vi "MENU8.vi"   [LabVIEW 2010, in "Lazyboots Menu Tool Launch.lvlib"]
uses:
  _Library/Lazyboots Menu Tool Launch.lvlib
  <vilib>/Utility/config.llb/Read Key (String).vi
  <vilib>/Utility/config.llb/NI_LVConfig.lvlib
panel:
  # "Launching..."
types:
  T1 = enum32{"Invalid", "Standard", "Closed", "Hidden", "Minimized", "Maximized"}
  T2 = typedef "NI_LVConfig.lvlib/Config Data RefNum.ctl" = refnum<k1>
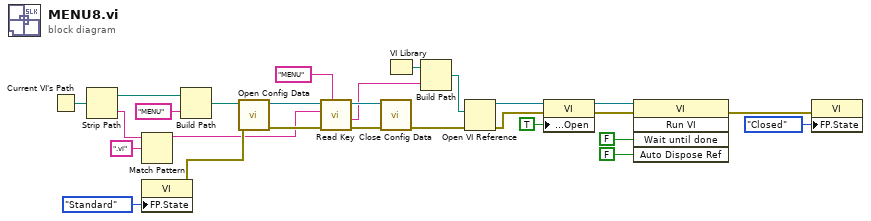
[diagram p0: block diagram]
diagram:
  n1 = Current VI's Path() -> (path=w25:path)
  n2 = Strip Path(path=w25) -> (stripped path=w24:path, name=w15:string)
  n3 = Match Pattern(string=w15, regular expression=".vi") -> (before substring=w14:string)  [unwired: 4 out]
  n4 = property class="VI"("FP.State"=T1."Standard" ("Front Panel Window:State")) -> (error out=w16:errorcluster)  [unwired: 2 in, 1 out]
  n5 = Build Path(base path=w24, name or relative path="MENU") -> (appended path=w22:path)
  n6 = call <vilib>:"Open Config Data.vi"("error in (no error)"=w16, "configuration file path"=w22) -> ("error out"=w20:errorcluster, "refnum"=w21:T2)  [unwired: 7 in, 1 out]
  n7 = call-poly <vilib>:"Read Key.vi"("section"="MENU", "error in (no error)"=w20, "key"=w14, "refnum"=w21) -> ("error out"=w17:errorcluster, "value"=w12:string, "refnum out"=w18:T2)  [unwired: 2 in, 3 out]
  n8 = call <vilib>:"Close Config Data.vi"("error in (no error)"=w17, "refnum"=w18) -> ("error out"=w3:errorcluster)  [unwired: 1 in, 8 out]
  n9 = VI Library() -> (path=w1:path)
  n10 = Build Path(base path=w1, name or relative path=w12) -> (appended path=w4:path)
  n11 = Open VI Reference(vi path=w4, error in (no error)=w3) -> (vi reference=w5:refnum<vi>, error out=w2:errorcluster)  [unwired: 4 in]
  n12 = property class="VI"(reference=w5, error in=w2, "Front Panel.Open"=TRUE ("Front Panel Window:Open")) -> (reference out=w8:refnum<vi>, error out=w7:errorcluster)
  n13 = invoke class="VI" method="Run VI"(reference=w8, error in=w7, "Wait until done"=FALSE ("Wait Until Done"), "Auto Dispose Ref"=FALSE ("Auto Dispose Reference")) -> (error out=w11:errorcluster)  [unwired: 1 in, 4 out]
  n14 = property class="VI"(error in=w11, "FP.State"=T1."Closed" ("Front Panel Window:State")) -> ()  [unwired: 1 in, 2 out]
